vi "Create New File.vi"(8 "error in":errorcluster, 10 "Path":path, 11 "TDMS File in":refnum<class "TDMS File.lvclass">) -> (0 "error out":errorcluster, 1 "path out":path, 2 "File Refnum":variant, 3 "TDMS File out":refnum<class "TDMS File.lvclass">)   [LabVIEW 2021, in "TDMS File.lvclass"]
doc: "This vi helps to create TDMS file and output a file reference as a variant."
uses:
  TDMS File.lvclass
  File Abstract Class/File Abstract.lvclass
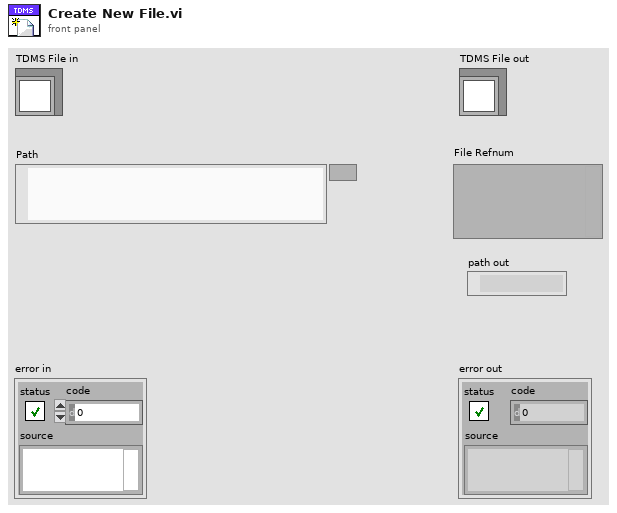
[diagram p1: front panel]
types:
  T1 = enum16{"open", "open or create", "create or replace", "create", "open (read-only)"}
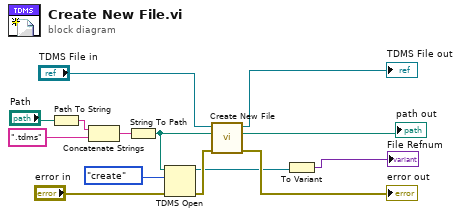
[diagram p0: block diagram]
diagram:
  n1 = Path To String(path="Path") -> (string=w2:string)
  n2 = Concatenate Strings(w2, ".tdms") -> (w4:string)
  n3 = String To Path(string=w4) -> (path=w3:path)
  "path out" <- w3
  n4 = TDMS Open(8:"error in", 10:T1."create" ("operation (0:open)"), 11:w3) -> (0:w9:errorcluster, 3:w7:refnum<k34>)  [unwired: 4 in]
  n5 = call-parent "Create New File.vi"("error in (no error)"=w9, "Path"=w3, "File Manager in"="TDMS File in") -> ("error out"=→"error out":errorcluster, "File Manager out"=→"TDMS File out":refnum<class "TDMS File.lvclass">)  [unwired: 5 in, 2 out]
  n6 = To Variant(anything=w7) -> (Variant=→"File Refnum":variant)
